vi "basic-start-stop-program.vi"() -> ()   [LabVIEW 2022 SP3]
uses:
  _driver/Basic driver/Communication/controls/comm_rate_enum.ctl
  _driver/_private/Control/Control Mode.ctl
  _driver/_private/Control/Programmable Mode.ctl
  <vilib>/Instr/_visa.llb/VISA Find Search Mode.ctl
  _driver/Chemyx_Syringe_Pump_driver.lvlib
panel:
  out "error out 2":errorcluster
  out "error out":errorcluster
  in  "error in (no error)":errorcluster
  in  "[x]":T1
  in  "Baud rate":T2
  in  "Com Port":string(combo)
  in  "Start":bool
  in  "Stop":bool
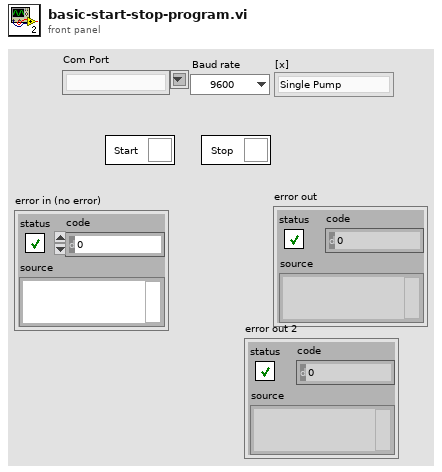
[diagram p1: front panel]
types:
  T1 = typedef "Chemyx_Syringe_Pump_driver.lvlib/Control Mode.ctl" = enum16{"Single Pump", "Pump Channel 1", "Pump Channel 2", "Cycle Mode"}
  T2 = typedef "Chemyx_Syringe_Pump_driver.lvlib/comm_rate_enum.ctl" = enum16{"9600", "38400"}
  T3 = typedef "VISA Find Search Mode.ctl" = u32
  T4 = typedef "Chemyx_Syringe_Pump_driver.lvlib/Programmable Mode.ctl" = enum16{"Blank", "Basic", "Programmable"}
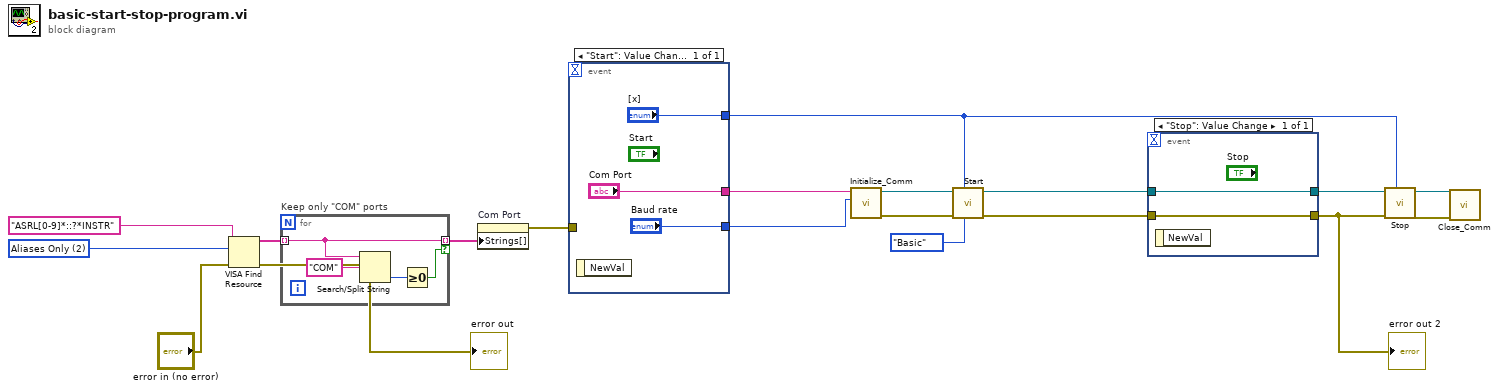
[diagram p0: block diagram]
diagram:
  w5 = T3 2 items=["Canonical Names Only"=0, "Aliases Only"=2, "Include Matching Aliases"=3, "Include All Aliases"=4] ("Search Mode")
  n1 = VISA Find Resource(8:"error in (no error)", 10:w5, 11:"ASRL[0-9]*::?*INSTR" ("expression (\"?*\")")) -> (0:→"error out":errorcluster, 3:w7:string[])  [unwired: 1 out]
  n2 = for "Keep only \"COM\" ports" {
    tunnel: w7 -> [w21] mode=indexing
    tunnel: [w21] -> w2 mode=indexing if=w20
    n3 = Search/Split String(string=w21, search string/char (-)="COM") -> (offset of match=w22:i32)  [unwired: 1 in, 2 out]
    n4 = Greater Or Equal To 0?(x=w22) -> (x >= 0?=w20:bool)
  }
  n5 = property on="Com Port" class="CmbBox"("Strings[]"=w2) -> (error out=w10:errorcluster)  [unwired: 2 in, 1 out]
  n6 = event shown="[0] \"Start\": Value Change" {
    selector: _ -> [_]
    dyn-events: _ -> [_]
    timeout: _ -> [_]
    tunnel: ["Com Port"] -> w19
    tunnel: ["Baud rate"] -> w11
    tunnel: w10 -> [_]
    tunnel: ["[x]"] -> w9
    event "Start": Value Change {
      n7 = event-data() -> ()  [unwired: 1 in, 1 out]
    }
  }
  n8 = call "Initialize_Comm.vi"("Baud rate"=w11, "Serial Port in"=w19) -> ("error out"=w15:errorcluster, "Serial Port out"=w16:refnum<visa-resource-name>)  [unwired: 8 in]
  n9 = call "Start.vi"("Mode"=Programmable_Mode."Basic", "[x]"=w9, "error in (no error)"=w15, "Serial Port in"=w16) -> ("error out"=w13:errorcluster, "Serial Port out"=w14:refnum<visa-resource-name>)  [unwired: 6 in]
  n10 = event shown="[0] \"Stop\": Value Change" {
    selector: _ -> [_]
    dyn-events: _ -> [_]
    timeout: _ -> [_]
    tunnel: [w28] -> w12
    tunnel: w14 -> [w28]
    tunnel: [w27] -> w1
    tunnel: w13 -> [w27]
    event "Stop": Value Change {
      n11 = event-data() -> ()  [unwired: 1 in, 1 out]
    }
  }
  "error out 2" <- w1
  n12 = call "Stop.vi"("[x]"=w9, "error in (no error)"=w1, "Serial Port in"=w12) -> ("error out"=w17:errorcluster, "Serial Port out"=w18:refnum<visa-resource-name>)  [unwired: 7 in]
  n13 = call "Close_Comm.vi"("error in (no error)"=w17, "Serial Port in"=w18) -> ()  [unwired: 9 in, 1 out]
